vi "updateAttributeTree_action.vi"(0 "HGF_ImaqDx":refnum<class "HGF_ImaqDx.lvclass">, 1 "Tree Control In":refnum<vi>, 3 "Flush Tree?":bool, 5 "error in (no error)":errorcluster) -> (14 "dup HGF_ImaqDx":refnum<class "HGF_ImaqDx.lvclass">, 15 "Tree Control Out":refnum<vi>, 19 "error out":errorcluster)   [LabVIEW 2014, in "HGF_IMAQ.lvlib" / "HGF_ImaqDx.lvclass"]
doc: "This is the override VI to update the referenced tree with cameras attribute names and values."
uses:
  HGF_ImaqDx.lvclass
  HGF_VisionTools/HGF_VisionTools.lvlib
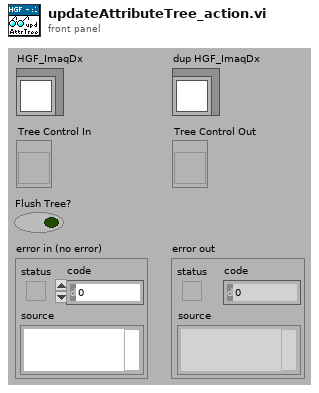
[diagram p1: front panel]
types:
  T1 = typedef "IMAQdx.ctl" = refnum<k21>
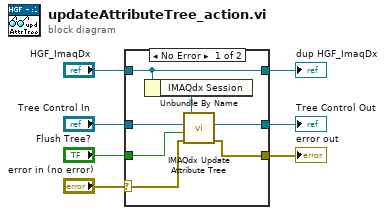
[diagram p0: block diagram]
diagram:
  n1 = case shown="No Error" "error in (no error)" {
    selector: "error in (no error)" -> [w9 w15]
    tunnel: "HGF_ImaqDx" -> [w8 w17]
    tunnel: "Tree Control In" -> [w14 w16]
    tunnel: "Flush Tree?" -> [w13 _]
    tunnel: [w12 w16] -> w4
    tunnel: [w10 w15] -> w3
    tunnel: [w8 w17] -> w1
    frame No Error {
      n2 = Unbundle By Name(w8) -> ("IMAQdx Session"=w11:T1)
      n3 = call "IMAQdx Update Attribute Tree.vi"("error in"=w9, "Flush Tree?"=w13, "Tree Control In"=w14, "Camera Name In"=w11) -> ("error out"=w10:errorcluster, "Tree Control Out"=w12:refnum<vi>)  [unwired: 1 in, 1 out]
    }
    frame Error {
    }
  }
  "error out" <- w3
  "dup HGF_ImaqDx" <- w1
  "Tree Control Out" <- w4
